vi "refMgr_Example4.vi"() -> ()   [LabVIEW 2017]
uses:
  40be52e9-3771-4604-be95-a9dd39ca470b.vi
  <userlib>/_NEVSTOP/TagDB/_Support/DataAccess/data-Write.vi
  <userlib>/_NEVSTOP/TagDB/_Support/Error/_[error50000]Invalid DB REF.vi
  <userlib>/_NEVSTOP/TagDB/_Support/DataAccess/TagDB Ref to DVR.vi
  <userlib>/_NEVSTOP/TagDB/_Support/DataAccess/_NameCacher.vi
  <userlib>/_NEVSTOP/TagDB/_Support/DataAccess/_datatypeChecker.vi
  <userlib>/_NEVSTOP/TagDB/_Support/Error/_Build Error Cluster.vi
  <vilib>/Utility/Data Type/Get Type Information.vi
  RefManager/_Support/UISync/_Publish DP Indicators(VI).vi
  <userlib>/_NEVSTOP/TagDB/TagDB.lvlib
  RefManager/TagDB RefManager.lvlib
panel:
  out "Numeric 3":dbl
  out "Numeric 4":dbl
  out "Numeric 8":dbl
  out "Numeric 9":dbl
  out "Numeric 6":dbl
  out "Numeric 5":dbl
  out "Numeric 1":dbl
  out "Numeric 0":dbl
  out "Numeric 7":dbl
  out "Numeric 2":dbl
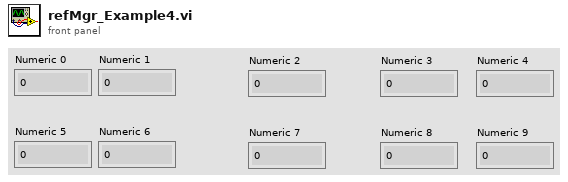
[diagram p1: front panel]
types:
  T1 = typedef "TagDB.lvlib/TagDB.ctl" = refnum<k1>
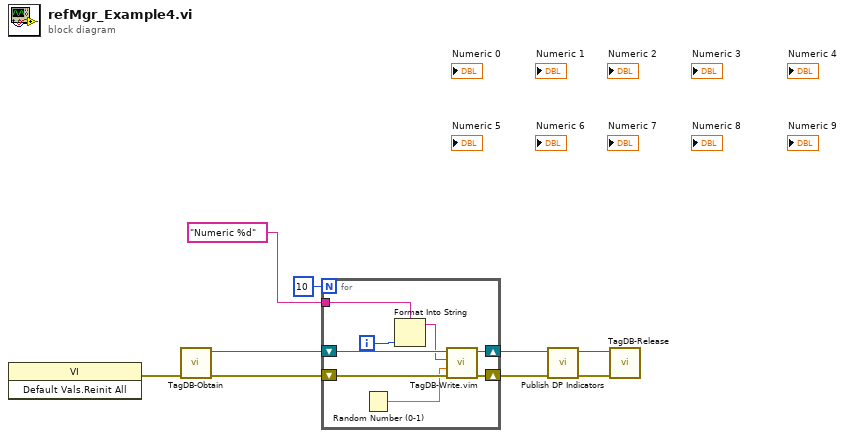
[diagram p0: block diagram]
diagram:
  n1 = invoke class="VI" method="Default Vals.Reinit All"() -> (error out=w8:errorcluster)  [unwired: 3 in, 2 out]
  n2 = call <userlib>:"TagDB-Obtain.vi"("error in (no error)"=w8) -> ("error out"=w6:errorcluster, "TagDB"=w9:T1)  [unwired: 4 in, 1 out]
  n3 = for {
    N: 10 -> [_]
    tunnel: "Numeric %d" ("name") -> [w13]
    shift-right: [w16] -> w5
    shift-left: w9 -> [w17]
    shift-right: [w10] -> w2
    shift-left: w6 -> [w15]
    i -> [w11]
    n4 = Random Number (0-1)() -> (number: 0 to 1=w12:dbl)
    n5 = Format Into String(format string=w13, w11) -> (resulting string=w14:string)  [unwired: 2 in, 1 out]
    n6 = call "TagDB-Write.vim"("error in (no error)"=w15, "Value"=w12, "name"=w14, "TagDB"=w17) -> ("error out"=w10:errorcluster, "TagDB(dup)"=w16:T1)  [unwired: 5 in, 1 out]
  }
  n7 = call-poly "Publish DP Indicators.vi"("error in (no error)"=w2, "SILAPI In"=w5) -> ("error out"=w1:errorcluster, "SILAPI Out"=w4:T1)  [unwired: 7 in, 1 out]
  n8 = call <userlib>:"TagDB-Release.vi"("error in (no error)"=w1, "TagDB"=w4) -> ()  [unwired: 9 in, 1 out]
